vi "MccHat_read.vi"(8 "error in":errorcluster, 11 "conn_id_in":refnum<k5>) -> (0 "error out":errorcluster, 2 "readings":cluster{i32, i32, dbl}[](array[cluster]), 3 "conn_id_out":refnum<k5>, 4 "status":bool)   [LabVIEW 2019]
panel:
  out "string_raw":string
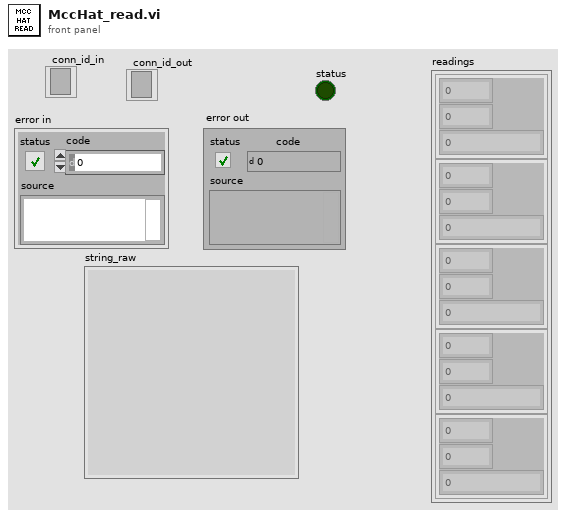
[diagram p1: front panel]
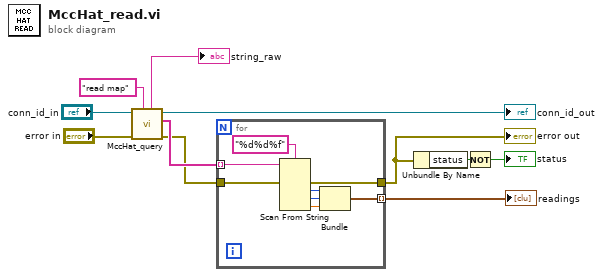
[diagram p0: block diagram]
diagram:
  n1 = call "MccHat_query.vi"("command"="read map" ("string"), "error in"="error in", "conn_id_in"="conn_id_in") -> ("error out"=w2:errorcluster, "string_array"=w4:string[], "conn_id_out"=→"conn_id_out":refnum<k5>, "string_raw"=→"string_raw":string)  [unwired: 4 in, 1 out]
  n2 = for {
    tunnel: w4 -> [w19] mode=indexing
    tunnel: [w14] -> w3 mode=indexing
    tunnel: w2 -> [w13]
    tunnel: [w12] -> w1
    n3 = Scan From String(format string="%d%d%f", input string=w19, error in=w13) -> (error out=w12:errorcluster, output 1=w17:i32, output 2=w16:i32, output 3=w15:dbl)  [unwired: 4 in, 2 out]
    n4 = Bundle(w17, w16, w15) -> (w14:cluster{i32, i32, dbl})  [unwired: 1 in]
  }
  "error out" <- w1
  "readings" <- w3
  n5 = Unbundle By Name(w1) -> ("status"=w6:bool)
  n6 = Not(x=w6) -> (.not. x?=→"status":bool)
